vi "turn(SubVI).vi"(8 "PID stuff":T1={"K Derivative"=0.000578344411839991, "K Proportional"=0.06728988505411036, "K Integral"=0.0}, 9 "setpoint PID":dbl) -> ()   [LabVIEW 2011]
uses:
  <vilib>/addons/control/pid/pid.llb/PID (DBL).vi
  <vilib>/addons/control/pid/NI_PID_pid.lvlib
panel:
  # "P: 0.0444, I: 0.00, D: 0.002929"
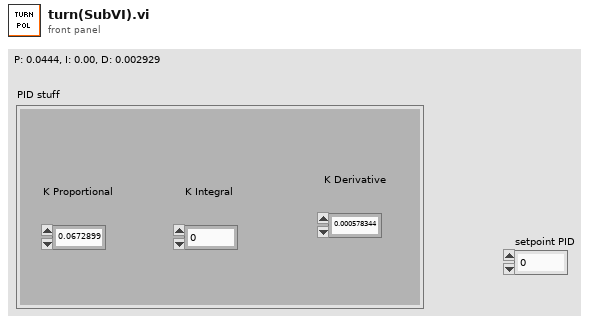
[diagram p1: front panel]
types:
  T1 = cluster{"K Derivative":dbl, "K Proportional":dbl, "K Integral":dbl}
  T2 = typedef "WPI_GyroDevRef.ctl" = cluster{"DevStatus":errorcluster, "Analog Module":T3, "Analog Channel":T4, "Offset":dbl, "Gain (VoltsPerDegree/Second)":dbl}
  T3 = typedef "FPGA_TypedefAnalogModule.ctl" = enum16{"Analog Module 1", "Analog Module 2"}
  T4 = typedef "FPGA_AIChannel.ctl" = enum8{"AI 1", "AI 2", "AI 3", "AI 4", "AI 5", "AI 6", "AI 7", "AI 8", "Invalid"}
  T5 = typedef "WPI_RobotDriveDevRef.ctl" = cluster{"DevStatus":errorcluster, "Motors[]":T6[], "Square Inputs":bool, "Max Output":dbl, "Isochronous":bool}
  T6 = typedef "WPI_MotorControlDeviceRef.ctl" = cluster{"DeviceStatus":errorcluster, "Type":enum16{"PWM", "CAN"}, "PWM":cluster{"Digital Module":T7, "PWM Channel":T8, "DeadBand":T9}, "CAN":cluster{"Device Number":u8, "Control Mode":T10, "Semaphore":T11, "Max Vout":dbl}, "Invert":bool, "TransformRef":T12, "InvTransformRef":T12}
  T7 = typedef "FPGA_TypedefDigitalModule.ctl" = enum16{"Digital Module 1", "Digital Module 2"}
  T8 = typedef "FPGA_DIOPWMChannel.ctl" = enum8{"PWM 1", "PWM 2", "PWM 3", "PWM 4", "PWM 5", "PWM 6", "PWM 7", "PWM 8", "PWM 9", "PWM 10", "Invalid"}
  T9 = typedef "WPI_PWMDeadband.ctl" = cluster{"Name":string, "maxPositivePwm":i32, "minPositivePwm":i32, "centerPwm":i32, "maxNegativePwm":i32, "minNegativePwm":i32, "angularRange":u16}
  T10 = typedef "WPI_CANJaguar_ControlMode.ctl" = enum8{"Percent VBus", "Current", "Speed", "Position", "Voltage"}
  T11 = typedef "Semaphore RefNum" = refnum<k1>
  T12 = typedef "WPI_PWMTransform_ConPane.ctl" = refnum<vi>
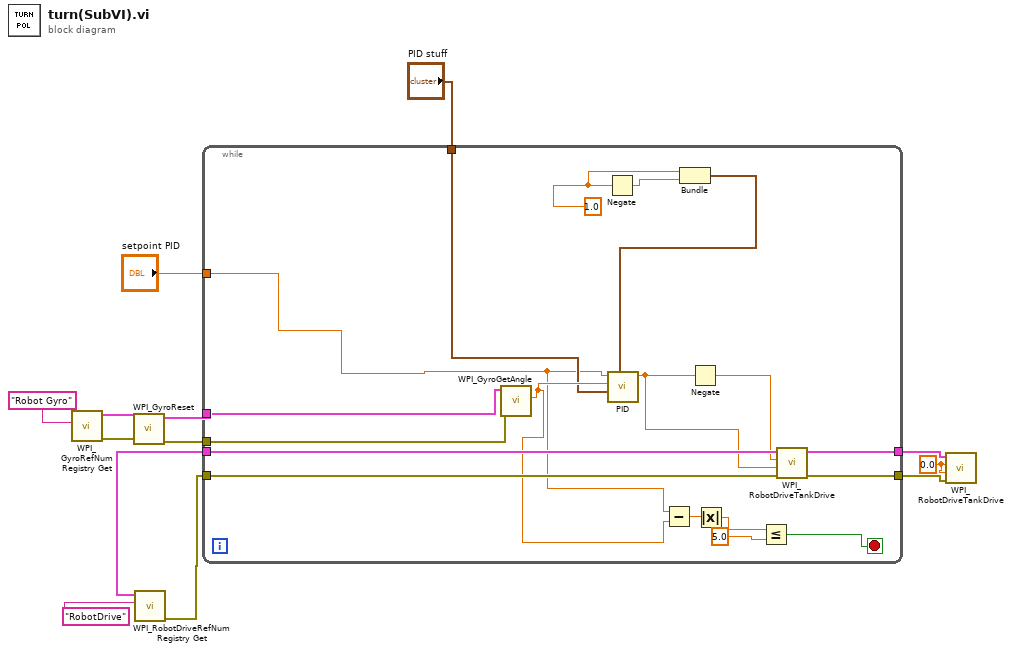
[diagram p0: block diagram]
diagram:
  w3 = 0.0 ("Left axis value")
  n1 = call <vilib>:"WPI_GyroRefNum Registry Get.vi"("refnum name"="Robot Gyro") -> ("error out"=w9:errorcluster, "GyroDevRef"=w10:T2)  [unwired: 9 in]
  n2 = call <vilib>:"WPI_GyroReset.vi"("error in (no error)"=w9, "GyroDevRef"=w10) -> ("error out"=w12:errorcluster, "GyroDevRef"=w13:T2)  [unwired: 8 in]
  n3 = call <vilib>:"WPI_RobotDriveRefNum Registry Get.vi"("refnum name"="RobotDrive") -> ("error out"=w8:errorcluster, "RobotDriveDevRef"=w7:T5)  [unwired: 9 in]
  n4 = while {
    tunnel: w13 -> [w31]
    tunnel: w12 -> [w30]
    tunnel: w7 -> [w29]
    tunnel: w8 -> [w28]
    tunnel: [w19] -> w5
    tunnel: [w18] -> w4
    tunnel: "setpoint PID" -> [w15]
    tunnel: "PID stuff" -> [w16]
    stop <- w14 stop-if-true
    w20 = 1.0 ("turn power")
    n5 = call <vilib>:"WPI_GyroGetAngle.vi"("error in (no error)"=w30, "GyroDevRef"=w31) -> ("Angle"=w17:dbl)  [unwired: 6 in, 3 out]
    n6 = Negate(x=w20) -> (-x=w22:dbl)
    n7 = Subtract(x=w15, y=w17) -> (x-y=w27:dbl)
    n8 = Bundle("turn power"=w20, w22) -> (w21:cluster{"turn power":dbl, dbl})  [unwired: 1 out]
    n9 = call-poly <vilib>:"PID.vi"("output range"=w21, "PID gains"=w16, "process variable"=w17, "setpoint"=w15) -> ("output"=w24:dbl)  [unwired: 6 in, 1 out]
    n10 = Negate(x=w24) -> (-x=w23:dbl)
    n11 = Absolute Value(x=w27) -> (abs(x)=w26:dbl)
    n12 = Less Or Equal?(x=w26, y=5.0) -> (x <= y?=w14:bool)
    n13 = call <vilib>:"WPI_RobotDriveTankDrive.vi"("error in (no error)"=w28, "Right axis value"=w24, "Left axis value"=w23, "RobotDriveDevRef"=w29) -> ("error out"=w18:errorcluster, "RobotDriveDevRef"=w19:T5)  [unwired: 6 out]
  }
  n14 = call <vilib>:"WPI_RobotDriveTankDrive.vi"("error in (no error)"=w4, "Right axis value"=w3, "Left axis value"=w3, "RobotDriveDevRef"=w5) -> ()  [unwired: 8 out]
